vi "Demo_SmartCam_GettingStart.vi"() -> ()   [LabVIEW 2017]
uses:
  IMAQCV/PIIO/Core/PIIO DIO.ctl
  IMAQCV/GPIO/GPIO Pins.ctl
  <vilib>/functionblocks/Edge Detection/One Shot Falling With Input/One Shot Falling With Input.vi
  <vilib>/functionblocks/FB Core/FB Core.xnode
  IMAQCV/IMAQCV.lvlib
  IMAQCV/PIIO.lvlib
  IMAQCV/LVOpenCV.lvlib
  <vilib>/functionblocks/NI_FunctionBlock Libraries.lvlib
  <vilib>/NI_Real-Time Target Support.lvlib
panel:
  in  "x df 10":i32=300
  in  "y df 10":i32=80
  out "output":bool
  in  "x df 9":i32=300
  in  "y df 9":i32=60
  in  "x df 8":i32=300
  in  "y df 8":i32=40
  in  "x df 7":i32=300
  in  "y df 7":i32=20
  in  "x df 6":i32=-100
  in  "y df 6":i32=350
  out "Effect No.":i32=22
  in  "x df 5":i32=300
  in  "y df 5":i32=-80
  in  "y df 4":i32
  in  "x df 4":i32=300
  in  "y df 3":i32=-20
  in  "x df 3":i32=300
  in  "y df 2":i32=-40
  in  "x df 2":i32=300
  in  "y df":i32=-60
  in  "x df":i32=300
  out "Status":bool=TRUE
  in  "Shutter":i32
  in  "Meter":enum16{"AVERAGE", "SPOT", "BACKLIT", "MATRIX"}(ring)
  in  "AWB":T1(ring)=enum."AUTO"
  in  "FPS":i32=60
  in  "Type":enum16{"GRAY", "COLOR"}(ring)=enum."COLOR"
  in  "Image Size":T2(ring)=enum."640 (H)   x  480 (V) "
  in  "stop":bool
  out "Loop Rate (Hz)":u32=9
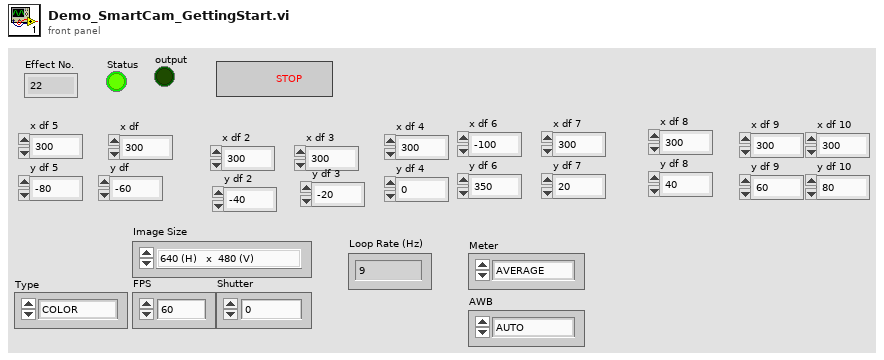
[diagram p1: front panel]
types:
  T1 = enum16{"OFF", "AUTO", "SUNLIGHT", "CLOUDY", "SHADE", "TUNGSTEN", "FLUORESCENT", "INCANDESCENT", "FLASH"}
  T2 = enum16{"320 (H)   x  240 (V)", "352(H)    x  288 (V)", "640 (H)   x  480 (V) ", "800 (H)   x  600 (V)", "1024 (H) x  768 (V)", "1280 (H) x  720 (V)", "1280 (H) x  960 (V)", "1280 (H) x 1024 (V)", "1920 (H) x 1080 (V)"}
  T3 = enum8{"INPUT", "OUTPUT", "PWM_OUTPUT", "GPIO_CLOCK", "SOFT_PWM_OUTPUT", "SOFT_TONE_OUTPUT", "PWM_TONE_OUTPUT"}
  T4 = cluster{"threshold1":i32, "threshold2":i32, "apertureSize":i32, "L2gradient":i8}
  T5 = enum16{"NONE", "NEGATIVE", "SOLARIZE", "SKETCH", "DENOISE", "EMBOSS", "OILPAINT", "HATCH", "GPEN", "PASTEL", "WATERCOLOR", "FILM", "BLUR", "SATURATION", "COLORSWAP", "WASHEDOUT", "POSTERISE", "COLORPOINT", "COLORBALANCE", "CARTOON"}
  T6 = typedef "PIIO.lvlib/GPIO Pins.ctl" = u8
  T7 = typedef "PIIO.lvlib/PIIO DIO.ctl" = u8
  T8 = typedef "IMAQCV.lvlib/IMAQCV Image.ctl" = refnum<vi>
  T9 = typedef "NI_Real-Time Target Support.lvlib/RT CPU Load.ctl" = cluster{"Total (%)":dbl, "Time Critical (%)":dbl, "Timed Structures (%)":dbl, "High (%)":dbl, "Above Normal (%)":dbl, "Normal (%)":dbl, "Background (%)":dbl, "Idle (%)":dbl, "ISR (%)":dbl}
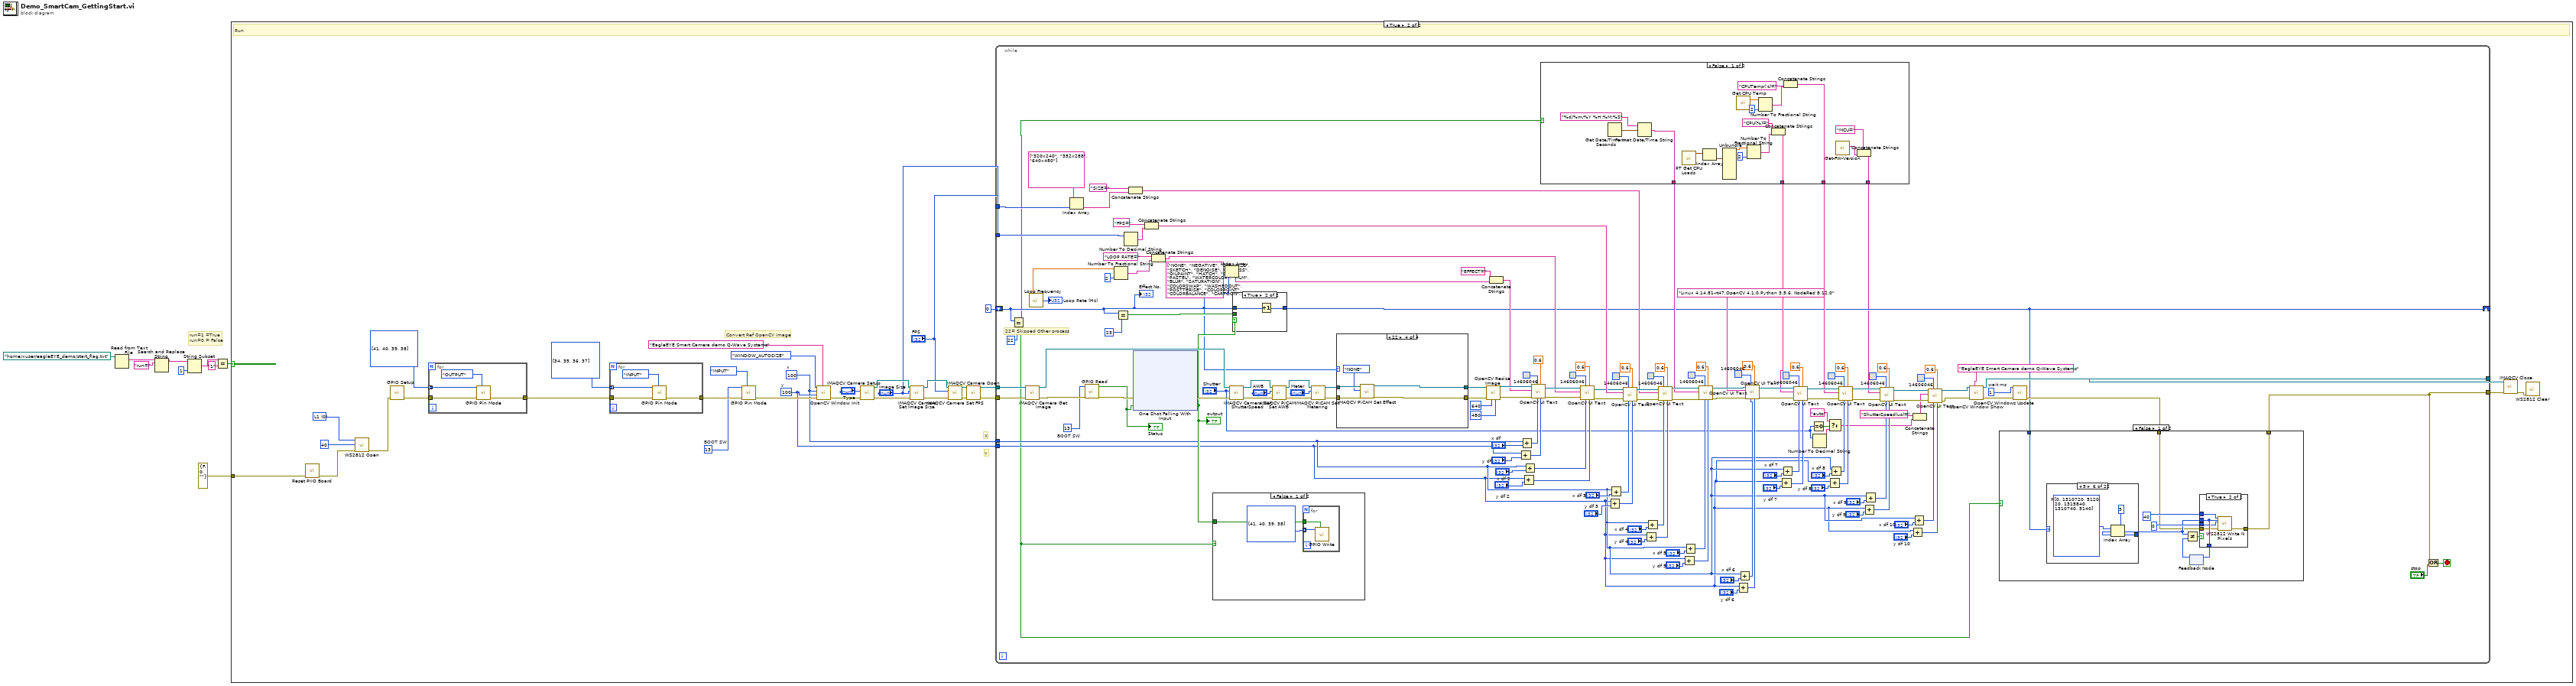
[diagram p0: block diagram]
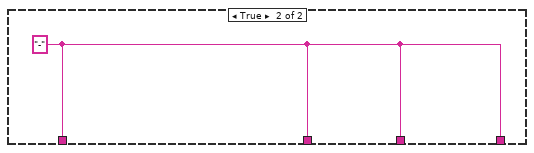
[diagram p4: hidden frame]
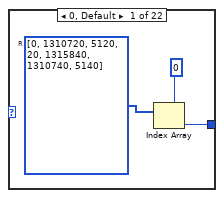
[diagram p5: hidden frame]
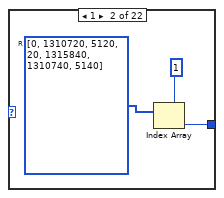
[diagram p6: hidden frame]
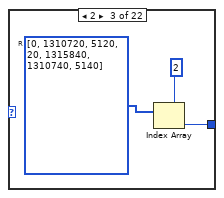
[diagram p7: hidden frame]
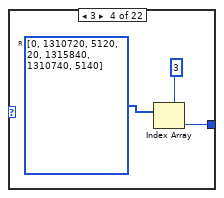
[diagram p8: hidden frame]
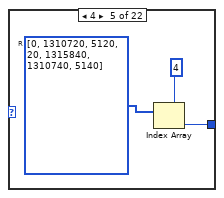
[diagram p9: hidden frame]
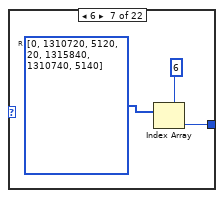
[diagram p10: hidden frame]
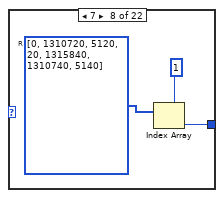
[diagram p11: hidden frame]
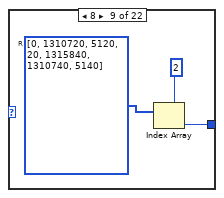
[diagram p12: hidden frame]
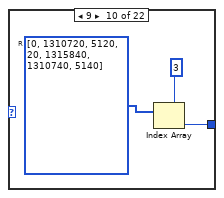
[diagram p13: hidden frame]
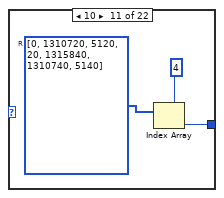
[diagram p14: hidden frame]
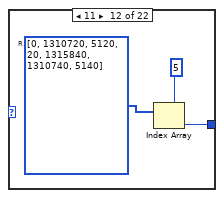
[diagram p15: hidden frame]
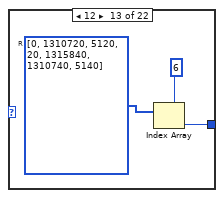
[diagram p16: hidden frame]
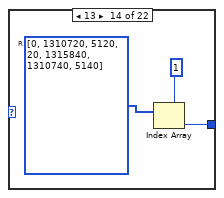
[diagram p17: hidden frame]
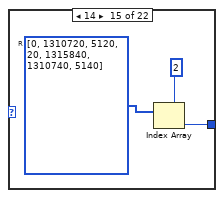
[diagram p18: hidden frame]
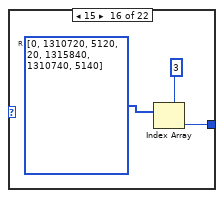
[diagram p19: hidden frame]
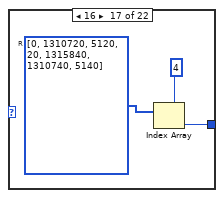
[diagram p20: hidden frame]
diagram:
  # "run=1 =True\nrun=0 = False"
  n1 = Read from Text File(file (use dialog)=path "/home/xuser/eagleEYE_demo/start_flag.txt") -> (text=w8:string)  [unwired: 3 in, 3 out]
  n2 = Search and Replace String(input string=w8, search string="run=") -> (result string=w4:string)  [unwired: 6 in, 3 out]
  n3 = String Subset(string=w4, length (rest)=1 ("length (rest)")) -> (substring=w3:string)  [unwired: 1 in]
  n4 = Equal?(x=w3, y="1") -> (x = y?=w6:bool)
  n5 = case shown="True" w6 {
    tunnel: errorcluster {"status"=FALSE, "code"=0, "source"=""} ("error in (no error)") -> [_ w10]
    frame False {
      # "Exit"
    }
    frame True {
      w11 = T6[] [34, 35, 36, 37] items=["DI-CH1"=34, "DI-CH2"=35, "DI-CH3"=36, "DI-CH4"=37, "DO-CH1"=41, "DO-CH2"=40, "DO-CH3"=39, "DO-CH4"=38]
      w12 = T6[] [41, 40, 39, 38] items=["DI-CH1"=34, "DI-CH2"=35, "DI-CH3"=36, "DI-CH4"=37, "DO-CH1"=41, "DO-CH2"=40, "DO-CH3"=39, "DO-CH4"=38]
      w13 = T7 0 items=["L1", "L2"] ("PIN")
      w25 = 13  # BOOT SW
      w22 = u32 100  # y
      w21 = u32 100  # x
      # "Y"
      # "X"
      # "Convert Ref OpenCV Image"
      # "Run"
      n6 = call "Reset PIIO Board.vi"("error in (no error)"=w10) -> ("error out"=w18:errorcluster)  [unwired: 10 in]
      n7 = call "WS2812 Open.vi"("Error In"=w18, "Number of LEDs"=u16 40, "PIN"=w13) -> ("Error Out"=w16:errorcluster)  [unwired: 8 in]
      n8 = call "GPIO Setup.vi"("error in (no error)"=w16) -> ("error out"=w29:errorcluster)  [unwired: 10 in]
      n9 = for {
        tunnel: w29 -> [w50]
        tunnel: [w49] -> w28
        tunnel: w12 -> [w47] mode=indexing
        n10 = call "GPIO Pin Mode.vi"("Pin Mode"=enum8{"INPUT", "OUTPUT"}."OUTPUT", "error in (no error)"=w50, "GPIO"=w47) -> ("error out"=w49:errorcluster)  [unwired: 8 in]
      }
      n11 = for {
        tunnel: w28 -> [w46]
        tunnel: [w45] -> w26
        tunnel: w11 -> [w43] mode=indexing
        n12 = call "GPIO Pin Mode.vi"("Pin Mode"=enum8{"INPUT", "OUTPUT"}."INPUT", "error in (no error)"=w46, "GPIO"=w43) -> ("error out"=w45:errorcluster)  [unwired: 8 in]
      }
      n13 = call "GPIO Pin Mode.vi"("Pin Mode"=T3."INPUT", "error in (no error)"=w26, "GPIO"=w25) -> ("error out"=w24:errorcluster)  [unwired: 8 in]
      n14 = call "OpenCV Window Init.vi"("window name"="EagleEYE Smart Camera demo Q-Wave Systems", "error in (no error)"=w24, "y"=w22, "x"=w21, "mode"=enum8{"WINDOW_AUTOSIZE", "WINDOW_FULLSCREEN"}."WINDOW_AUTOSIZE") -> ("error out"=w31:errorcluster)  [unwired: 6 in]
      n15 = call "IMAQCV Camera Setup.vi"("error in (no error)"=w31, "type"="Type") -> ("error out"=w42:errorcluster, "image out"=w41:T8)  [unwired: 8 in]
      n16 = call "IMAQCV Camera Set Image Size.vi"("error in (no error)"=w42, "Image Size"="Image Size", "image in"=w41) -> ("error out"=w37:errorcluster, "image out"=w36:T8)  [unwired: 7 in]
      n17 = call "IMAQCV Camera Set FPS.vi"("error in (no error)"=w37, "FPS"="FPS", "image in"=w36) -> ("error out"=w34:errorcluster, "image out"=w35:T8)  [unwired: 7 in]
      n18 = call "IMAQCV Camera Open.vi"("error in (no error)"=w34, "image in"=w35) -> ("error out"=w40:errorcluster, "image out"=w39:T8)  [unwired: 8 in]
      n19 = while {
        tunnel: w39 -> [w198]
        tunnel: w40 -> [w181]
        tunnel: [w184] -> w30
        shift-right: [w85] -> _
        shift-left: 0 -> [w53]
        tunnel: w22 -> [w55]
        tunnel: w21 -> [w56]
        tunnel: "FPS" -> [w167]
        tunnel: "Image Size" -> [w139]
        tunnel: [w86] -> w14
        stop <- w199 stop-if-true
        w51 = 13  # BOOT SW
        w187 = 1  # wait ms
        # "22= Skipped Other process"
        n20 = Equal?(x=w53, y=22) -> (x = y?=w52:bool)
        n21 = call "IMAQCV Camera Get Image.vi"("error in (no error)"=w181, "image in"=w198) -> ("error out"=w75:errorcluster, "image out"=w191:T8)  [unwired: 8 in]
        n22 = call "Loop Frequency.vi"() -> ("Loop Rate (Hz)"=→"Loop Rate (Hz)":u32, "Loop Rate (Hz) DBL"=w143:dbl)
        n23 = Index Array(array=string[] ["320x240", "352x288", "640x480"], index=w139) -> (element=w138:string)
        n24 = call "GPIO Read.vi"("error in (no error)"=w75, "GPIO"=w51) -> ("error out"=w178:errorcluster, "Status"=w74:bool)  [unwired: 8 in]
        "Status" <- w74
        n25 = Number To Fractional String(number=w143, precision (6)=i16 2) -> (F-format string=w145:string)  [unwired: 2 in]
        n26 = Equal?(x=w53, y=23) -> (x = y?=w179:bool)
        n27 = Number To Decimal String(number=w167) -> (decimal integer string=w164:string)  [unwired: 1 in]
        n28 = Concatenate Strings("SIZE=", w138) -> (w133:string)
        n29 = xnode "One Shot Falling With Input"("error in"=w178, "input"=w74) -> ("error out"=w177:errorcluster, "output"=w142:bool)
        "output" <- w142
        n30 = Concatenate Strings("FPS=", w164) -> (w160:string)
        n31 = Concatenate Strings("LOOP RATE=", w145) -> (w161:string)
        n32 = case shown="False" w52 {
          tunnel: w142 -> [w202 _]
          frame False {
            w201 = T6[] [41, 40, 39, 38] items=["DI-CH1"=34, "DI-CH2"=35, "DI-CH3"=36, "DI-CH4"=37, "DO-CH1"=41, "DO-CH2"=40, "DO-CH3"=39, "DO-CH4"=38]
            n33 = for {
              tunnel: w202 -> [w204]
              tunnel: w201 -> [w203] mode=indexing
              n34 = call "GPIO Write.vi"("Value"=w204, "GPIO"=w203) -> ()  [unwired: 9 in, 1 out]
            }
          }
          frame True {
          }
        }
        n35 = Index Array(array=string[] ["NONE", "NEGATIVE", "SOLARIZE", "SKETCH", "DENOISE", "EMBOSS", "OILPAINT", "HATCH", "GPEN", "PASTEL", "WATERCOLOR", "FILM", "BLUR", "SATURATION", "COLORSWAP", "WASHEDOUT", "POSTTERISE", "COLORPOINT", "COLORBALANCE", "CARTOON", "CANNY", "FACE_DETECT", "NONE-FAST"], index=w53) -> (element=w127:string)
        n36 = call "IMAQCV Camera Set ShutterSpeed.vi"("error in (no error)"=w177, "shutter speed (us, 0=auto)"="Shutter", "image in"=w191) -> ("error out"=w183:errorcluster, "image out"=w182:T8)  [unwired: 7 in]
        n37 = case shown="True" w142 {
          tunnel: w53 -> [w374 w378]
          tunnel: [w375 w377] -> w85
          tunnel: w179 -> [w373 _]
          frame False {
            n38 = Select(t=0 ("y"), s=w373, f=w374) -> (s? t:f=w375:i32)
          }
          frame True {
            n39 = Increment(x=w378) -> (x+1=w377:i32)
          }
        }
        n40 = call "IMAQCV PiCAM Set AWB.vi"("error in (no error)"=w183, "AWB"="AWB", "image in"=w182) -> ("error out"=w196:errorcluster, "image out"=w194:T8)  [unwired: 7 in]
        n41 = call "IMAQCV PiCAM Set Metering.vi"("error in (no error)"=w196, "mode"="Meter", "image in"=w194) -> ("error out"=w195:errorcluster, "image out"=w193:T8)  [unwired: 7 in]
        n42 = case shown="22" w53 {
          selector: w53 -> [w307 _ _ _]
          tunnel: w195 -> [w311 w319 w329 w334]
          tunnel: w193 -> [w310 w318 w328 w333]
          tunnel: [w309 w321 w325 w331] -> w186
          tunnel: [w308 w322 w324 w330] -> w185
          frame 0, Default {
            n43 = call "IMAQCV PiCAM Set Effect.vi"("error in (no error)"=w311, "effect"=w307, "image in"=w310) -> ("error out"=w309:errorcluster, "image out"=w308:T8)  [unwired: 7 in]
          }
          frame 20 {
            w316 = u32 6 items=["RGB (U32)"=0, "Grayscale (U8)"=6, "RGB-Grayscale (U8)"=10, "Gray-RGB (U32)"=9] ("code")
            n44 = call "IMAQCV PiCAM Set Effect.vi"("error in (no error)"=w319, "effect"=T5."NONE", "image in"=w318) -> ("error out"=w315:errorcluster, "image out"=w314:T8)  [unwired: 7 in]
            n45 = call "OpenCV cvtColor.vi"("error in (no error)"=w315, "code"=w316, "image in"=w314) -> ("error out"=w312:errorcluster, "image out"=w313:T8)  [unwired: 7 in]
            n46 = call "OpenCV Canny.vi"("error in (no error)"=w312, "Canny Options"=T4 {"threshold1"=50, "threshold2"=50, "apertureSize"=3, "L2gradient"=-2}, "image"=w313) -> ("error out"=w321:errorcluster, "image out"=w322:T8)  [unwired: 7 in]
          }
          frame 21 {
            n47 = call "IMAQCV PiCAM Set Effect.vi"("error in (no error)"=w329, "effect"=T5."NONE", "image in"=w328) -> ("error out"=w326:errorcluster, "image out"=w323:T8)  [unwired: 7 in]
            n48 = call "FaceDetect_SubVI.vi"("error in (no error)"=w326, "image"=w323) -> ("error out"=w325:errorcluster, "image out"=w324:T8)  [unwired: 8 in]
          }
          frame 22 {
            n49 = call "IMAQCV PiCAM Set Effect.vi"("error in (no error)"=w334, "effect"=T5."NONE", "image in"=w333) -> ("error out"=w331:errorcluster, "image out"=w330:T8)  [unwired: 7 in]
          }
        }
        n50 = call "OpenCV Resize Image.vi"("height"=u32 480, "width"=u32 640, "error in (no error)"=w186, "image in"=w185) -> ("error out"=w175:errorcluster, "image out"=w176:T8)  [unwired: 6 in]
        n51 = Concatenate Strings("EFFECT=", w127) -> (w126:string)
        n52 = Add(x=w55, y="y df") -> (x+y=w173:u32)
        n53 = Add(x=w56, y="x df") -> (x+y=w174:u32)
        n54 = Add(x=w55, y="y df 2") -> (x+y=w146:u32)
        n55 = Add(x=w56, y="x df 2") -> (x+y=w147:u32)
        n56 = call "OpenCV UI Text.vi"("y"=w173, "font scale"=0.6, "x"=w174, "text color"=u32 14606046, "error in (no error)"=w175, "text"=w126, "image in"=w176) -> ("error out"=w163:errorcluster, "image out"=w162:T8)  [unwired: 3 in]
        n57 = case shown="False" w52 {
          tunnel: [w220 w223] -> w117
          tunnel: [w210 w223] -> w97
          tunnel: [w209 w223] -> w96
          tunnel: [w206 w223] -> w76
          frame False {
            n58 = Get Date/Time In Seconds() -> (seconds since 1Jan1904=w222:timestamp)
            n59 = Format Date/Time String(time format string (%c)="%d/%m/%Y %H:%M:%S", seconds (now)=w222) -> (date/time string=w220:string)  [unwired: 1 in]
            n60 = call <vilib>:"RT Get CPU Loads.vi"() -> ("CPU loads"=w205:T9[])  [unwired: 10 in, 1 out]
            n61 = Index Array(array=w205) -> (element=w219:T9)  [unwired: 1 in]
            n62 = Unbundle(w219) -> ("Total (%)"=w218:dbl)  [unwired: 8 out]
            n63 = call "Get CPU Temp.vi"() -> ("temp (C)"=w211:dbl)  [unwired: 10 in, 1 out]
            n64 = Number To Fractional String(number=w218, precision (6)=i16 2) -> (F-format string=w215:string)  [unwired: 2 in]
            n65 = Number To Fractional String(number=w211, precision (6)=i16 2) -> (F-format string=w214:string)  [unwired: 2 in]
            n66 = Concatenate Strings("CPU(%)=", w215) -> (w210:string)
            n67 = Concatenate Strings("CPUTemp('c)=", w214) -> (w209:string)
            n68 = call "Get-FW-Version.vi"() -> ("String"=w207:string)  [unwired: 9 in, 2 out]
            n69 = Concatenate Strings("MCU=" ("string"), w207) -> (w206:string)
          }
          frame True {
            w223 = "-"
          }
        }
        n70 = call "OpenCV UI Text.vi"("y"=w146, "font scale"=0.6, "x"=w147, "text color"=u32 14606046, "error in (no error)"=w163, "text"=w161, "image in"=w162) -> ("error out"=w159:errorcluster, "image out"=w158:T8)  [unwired: 3 in]
        n71 = Add(x=w55, y="y df 3") -> (x+y=w148:u32)
        n72 = Add(x=w56, y="x df 3") -> (x+y=w149:u32)
        n73 = call "OpenCV UI Text.vi"("y"=w148, "font scale"=0.6, "x"=w149, "text color"=u32 14606046, "error in (no error)"=w159, "text"=w160, "image in"=w158) -> ("error out"=w135:errorcluster, "image out"=w134:T8)  [unwired: 3 in]
        n74 = Add(x=w55, y="y df 4") -> (x+y=w129:u32)
        n75 = Add(x=w56, y="x df 4") -> (x+y=w130:u32)
        n76 = call "OpenCV UI Text.vi"("y"=w129, "font scale"=0.6, "x"=w130, "text color"=u32 14606046, "error in (no error)"=w135, "text"=w133, "image in"=w134) -> ("error out"=w123:errorcluster, "image out"=w122:T8)  [unwired: 3 in]
        n77 = Add(x=w55, y="y df 5") -> (x+y=w118:u32)
        n78 = Add(x=w56, y="x df 5") -> (x+y=w119:u32)
        n79 = call "OpenCV UI Text.vi"("y"=w118, "font scale"=0.6, "x"=w119, "text color"=u32 14606046, "error in (no error)"=w123, "text"=w117, "image in"=w122) -> ("error out"=w112:errorcluster, "image out"=w111:T8)  [unwired: 3 in]
        n80 = Add(x=w55, y="y df 6") -> (x+y=w107:u32)
        n81 = Add(x=w56, y="x df 6") -> (x+y=w108:u32)
        n82 = call "OpenCV UI Text.vi"("y"=w107, "font scale"=0.6, "x"=w108, "text color"=u32 14606046, "error in (no error)"=w112, "text"="Linux 4.14.81-rt47,OpenCV 4.1.0,Python 3.5.6, NodeRed 8.12.0", "image in"=w111) -> ("error out"=w101:errorcluster, "image out"=w98:T8)  [unwired: 3 in]
        n83 = Add(x=w55, y="y df 7") -> (x+y=w90:u32)
        n84 = Add(x=w56, y="x df 7") -> (x+y=w91:u32)
        n85 = call "OpenCV UI Text.vi"("y"=w90, "font scale"=0.6, "x"=w91, "text color"=u32 14606046, "error in (no error)"=w101, "text"=w97, "image in"=w98) -> ("error out"=w100:errorcluster, "image out"=w99:T8)  [unwired: 3 in]
        n86 = Equal To 0?(x="Shutter") -> (x = 0?=w65:bool)
        n87 = Number To Decimal String(number="Shutter") -> (decimal integer string=w63:string)  [unwired: 1 in]
        n88 = Select(t="auto", s=w65, f=w63) -> (s? t:f=w62:string)
        n89 = Add(x=w55, y="y df 8") -> (x+y=w88:u32)
        n90 = Add(x=w56, y="x df 8") -> (x+y=w89:u32)
        n91 = call "OpenCV UI Text.vi"("y"=w88, "font scale"=0.6, "x"=w89, "text color"=u32 14606046, "error in (no error)"=w100, "text"=w96, "image in"=w99) -> ("error out"=w82:errorcluster, "image out"=w81:T8)  [unwired: 3 in]
        n92 = Add(x=w55, y="y df 9") -> (x+y=w77:u32)
        n93 = Add(x=w56, y="x df 9") -> (x+y=w78:u32)
        n94 = call "OpenCV UI Text.vi"("y"=w77, "font scale"=0.6, "x"=w78, "text color"=u32 14606046, "error in (no error)"=w82, "text"=w76, "image in"=w81) -> ("error out"=w71:errorcluster, "image out"=w68:T8)  [unwired: 3 in]
        n95 = Add(x=w55, y="y df 10") -> (x+y=w57:u32)
        n96 = Add(x=w56, y="x df 10") -> (x+y=w58:u32)
        n97 = Concatenate Strings("ShutterSpeed(us)=", w62) -> (w66:string)
        n98 = call "OpenCV UI Text.vi"("y"=w57, "font scale"=0.6, "x"=w58, "text color"=u32 14606046, "error in (no error)"=w71, "text"=w66, "image in"=w68) -> ("error out"=w70:errorcluster, "image out"=w69:T8)  [unwired: 3 in]
        n99 = call "OpenCV Window Show.vi"("window name"="EagleEYE Smart Camera demo Q-Wave Systems", "error in (no error)"=w70, "image in"=w69) -> ("error out"=w190:errorcluster, "image out"=w184:T8)  [unwired: 7 in]
        n100 = call "OpenCV Windows Update.vi"("error in (no error)"=w190, "wait ms"=w187) -> ("error out"=w87:errorcluster)  [unwired: 8 in, 1 out]
        n101 = case shown="False" w52 {
          tunnel: w87 -> [w226 w306]
          tunnel: [w225 w306] -> w86
          tunnel: w85 -> [w224 _]
          frame False {
            n102 = case shown="5" w224 {
              tunnel: [w233 w236 w239 w242 w245 w248 w251 w254 w257 w260 w263 w266 w269 w272 w275 w278 w281 w284 w287 w290 w293 w296] -> w227
              frame 0, Default {
                # "GB"
                # "RB"
                # "RG"
                # "B"
                # "G"
                # "R"
                n103 = Index Array(array=u32[] [0, 1310720, 5120, 20, 1315840, 1310740, 5140] ("Array"), index=0) -> (element=w233:u32)
              }
              frame 1 {
                # "GB"
                # "RB"
                # "RG"
                # "B"
                # "G"
                # "R"
                n104 = Index Array(array=u32[] [0, 1310720, 5120, 20, 1315840, 1310740, 5140] ("Array"), index=1) -> (element=w236:u32)
              }
              frame 2 {
                # "GB"
                # "RB"
                # "RG"
                # "B"
                # "G"
                # "R"
                n105 = Index Array(array=u32[] [0, 1310720, 5120, 20, 1315840, 1310740, 5140] ("Array"), index=2) -> (element=w239:u32)
              }
              frame 3 {
                # "GB"
                # "RB"
                # "RG"
                # "B"
                # "G"
                # "R"
                n106 = Index Array(array=u32[] [0, 1310720, 5120, 20, 1315840, 1310740, 5140] ("Array"), index=3) -> (element=w242:u32)
              }
              frame 4 {
                # "GB"
                # "RB"
                # "RG"
                # "B"
                # "G"
                # "R"
                n107 = Index Array(array=u32[] [0, 1310720, 5120, 20, 1315840, 1310740, 5140] ("Array"), index=4) -> (element=w245:u32)
              }
              frame 5 {
                # "GB"
                # "RB"
                # "RG"
                # "B"
                # "G"
                # "R"
                n108 = Index Array(array=u32[] [0, 1310720, 5120, 20, 1315840, 1310740, 5140] ("Array"), index=5) -> (element=w248:u32)
              }
              frame 6 {
                # "GB"
                # "RB"
                # "RG"
                # "B"
                # "G"
                # "R"
                n109 = Index Array(array=u32[] [0, 1310720, 5120, 20, 1315840, 1310740, 5140] ("Array"), index=6) -> (element=w251:u32)
              }
              frame 7 {
                # "GB"
                # "RB"
                # "RG"
                # "B"
                # "G"
                # "R"
                n110 = Index Array(array=u32[] [0, 1310720, 5120, 20, 1315840, 1310740, 5140] ("Array"), index=1) -> (element=w254:u32)
              }
              frame 8 {
                # "GB"
                # "RB"
                # "RG"
                # "B"
                # "G"
                # "R"
                n111 = Index Array(array=u32[] [0, 1310720, 5120, 20, 1315840, 1310740, 5140] ("Array"), index=2) -> (element=w257:u32)
              }
              frame 9 {
                # "GB"
                # "RB"
                # "RG"
                # "B"
                # "G"
                # "R"
                n112 = Index Array(array=u32[] [0, 1310720, 5120, 20, 1315840, 1310740, 5140] ("Array"), index=3) -> (element=w260:u32)
              }
              frame 10 {
                # "GB"
                # "RB"
                # "RG"
                # "B"
                # "G"
                # "R"
                n113 = Index Array(array=u32[] [0, 1310720, 5120, 20, 1315840, 1310740, 5140] ("Array"), index=4) -> (element=w263:u32)
              }
              frame 11 {
                # "GB"
                # "RB"
                # "RG"
                # "B"
                # "G"
                # "R"
                n114 = Index Array(array=u32[] [0, 1310720, 5120, 20, 1315840, 1310740, 5140] ("Array"), index=5) -> (element=w266:u32)
              }
              frame 12 {
                # "GB"
                # "RB"
                # "RG"
                # "B"
                # "G"
                # "R"
                n115 = Index Array(array=u32[] [0, 1310720, 5120, 20, 1315840, 1310740, 5140] ("Array"), index=6) -> (element=w269:u32)
              }
              frame 13 {
                # "GB"
                # "RB"
                # "RG"
                # "B"
                # "G"
                # "R"
                n116 = Index Array(array=u32[] [0, 1310720, 5120, 20, 1315840, 1310740, 5140] ("Array"), index=1) -> (element=w272:u32)
              }
              frame 14 {
                # "GB"
                # "RB"
                # "RG"
                # "B"
                # "G"
                # "R"
                n117 = Index Array(array=u32[] [0, 1310720, 5120, 20, 1315840, 1310740, 5140] ("Array"), index=2) -> (element=w275:u32)
              }
              frame 15 {
                # "GB"
                # "RB"
                # "RG"
                # "B"
                # "G"
                # "R"
                n118 = Index Array(array=u32[] [0, 1310720, 5120, 20, 1315840, 1310740, 5140] ("Array"), index=3) -> (element=w278:u32)
              }
              frame 16 {
                # "GB"
                # "RB"
                # "RG"
                # "B"
                # "G"
                # "R"
                n119 = Index Array(array=u32[] [0, 1310720, 5120, 20, 1315840, 1310740, 5140] ("Array"), index=4) -> (element=w281:u32)
              }
              frame 17 {
                # "GB"
                # "RB"
                # "RG"
                # "B"
                # "G"
                # "R"
                n120 = Index Array(array=u32[] [0, 1310720, 5120, 20, 1315840, 1310740, 5140] ("Array"), index=5) -> (element=w284:u32)
              }
              frame 18 {
                # "GB"
                # "RB"
                # "RG"
                # "B"
                # "G"
                # "R"
                n121 = Index Array(array=u32[] [0, 1310720, 5120, 20, 1315840, 1310740, 5140] ("Array"), index=6) -> (element=w287:u32)
              }
              frame 19 {
                # "GB"
                # "RB"
                # "RG"
                # "B"
                # "G"
                # "R"
                n122 = Index Array(array=u32[] [0, 1310720, 5120, 20, 1315840, 1310740, 5140] ("Array"), index=1) -> (element=w290:u32)
              }
              frame 20 {
                # "GB"
                # "RB"
                # "RG"
                # "B"
                # "G"
                # "R"
                n123 = Index Array(array=u32[] [0, 1310720, 5120, 20, 1315840, 1310740, 5140] ("Array"), index=2) -> (element=w293:u32)
              }
              frame 21 {
                # "GB"
                # "RB"
                # "RG"
                # "B"
                # "G"
                # "R"
                n124 = Index Array(array=u32[] [0, 1310720, 5120, 20, 1315840, 1310740, 5140] ("Array"), index=3) -> (element=w296:u32)
              }
            }
            n125 = feedback #1() -> (w230:u32)  [unwired: 1 in]
            n126 = Not Equal?(x=w227, y=w230) -> (x != y?=w232:bool)
            n127 = case shown="True" w232 {
              tunnel: [w299 w305] -> w225
              tunnel: w227 -> [w300 w304]
              tunnel: [w300 w304] -> w231
              tunnel: u16 40 ("Number of LEDs") -> [_ w303]
              tunnel: u16 0 ("Start Pixel Index") -> [_ w302]
              tunnel: w226 -> [w299 w301]
              frame False {
              }
              frame True {
                n128 = call "WS2812 Write N Pixels.vi"("LED Color"=w304, "Error In"=w301, "Start Pixel Index"=w302, "Number of LEDs"=w303) -> ("Error Out"=w305:errorcluster)  [unwired: 7 in]
              }
            }
            n129 = feedback-in #1(w231) -> ()
          }
          frame True {
          }
        }
        n130 = Or(x=w86, y="stop") -> (x .or. y?=w199:bool)
        "Effect No." <- w53
      }
      n131 = call "IMAQCV Close.vi"("error in (no error)"=w14, "Image"=w30) -> ("error out"=w15:errorcluster)  [unwired: 9 in]
      n132 = call "WS2812 Clear.vi"("Error In"=w15) -> ()  [unwired: 10 in, 1 out]
    }
  }
